vi "_TangoAttributeConfigEventGroupCreate.vi"(0 "error in":errorcluster) -> (1 "attribute config event ref":T1, 2 "error out":errorcluster)   [LabVIEW 2014, in "tango.lvlib"]
uses:
  tango.lvlib
  Common VIs/Typedefs/_AttributeConfigEventRef.ctl
  Common VIs/Typedefs/_AttributeInfo_t.ctl
  Common VIs/Typedefs/_AttributeAccess_t.ctl
  Common VIs/Typedefs/_AttributeFormat_t.ctl
  Common VIs/Typedefs/_TangoDataType_t.ctl
  Common VIs/Typedefs/_AttributeLevel_t.ctl
  tango_binding.so
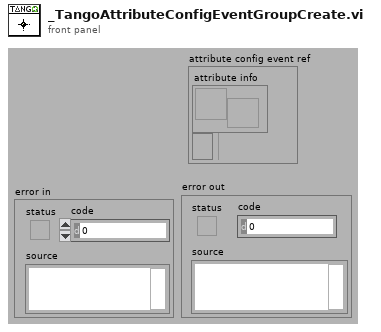
[diagram p1: front panel]
types:
  T1 = typedef "tango.lvlib/_AttributeConfigEventRef.ctl" = cluster{"attribute info":refnum<user-event>, "Event Registration Refnum":refnum<event-registration>}
  T2 = typedef "tango.lvlib/_AttributeInfo_t.ctl" = cluster{"device name":string, "attribute name":string, "r/w access":T3, "format":T4, "data type":T5, "level":T6, "label":string, "unit":string, "display format":string, "min value":string, "max value":string, "min alarm":string, "max alarm":string}
  T3 = typedef "tango.lvlib/_AttributeAccess_t.ctl" = enum16{"READ", "READ_WITH_WRITE", "WRITE", "READ_WRITE", "UNKNOWN_ACCESS_TYPE"}
  T4 = typedef "tango.lvlib/_AttributeFormat_t.ctl" = enum16{"SCALAR", "SPECTRUM", "IMAGE", "UNKNOWN_FORMAT"}
  T5 = typedef "tango.lvlib/_TangoDataType_t.ctl" = enum16{"VOID", "BOOLEAN", "SHORT", "LONG", "FLOAT", "DOUBLE", "USHORT", "ULONG", "STRING", "CHAR_ARRAY", "SHORT_ARRAY", "LONG_ARRAY", "FLOAT_ARRAY", "DOUBLE_ARRAY", "USHORT_ARRAY", "ULONG_ARRAY", "STRING_ARRAY", "LONG_STRING_ARRAY", "DOUBLE_STRING_ARRAY", "STATE", "CONST_STRING", "BOOLEAN_ARRAY", "UCHAR", "LONG64", "ULONG64", "LONG64_ARRAY", "ULONG64_ARRAY", "INT (not supported)", "ENCODED (not supported)", "ENUM", "PIPE_BLOB (not supported)", "STATE_ARRAY", "UNKNOW_DATA_TYPE"}
  T6 = typedef "tango.lvlib/_AttributeLevel_t.ctl" = enum16{"OPERATOR", "EXPERT", "UNKNOWN_LEVEL"}
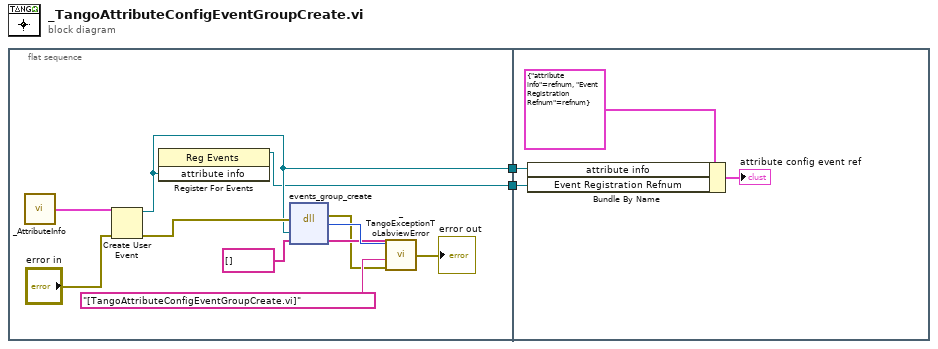
[diagram p0: block diagram]
diagram:
  n1 = flat-sequence {
    tunnel: [w5] -> w2
    tunnel: [w4] -> w1
    tunnel: w2 -> [w17]
    tunnel: w1 -> [w16]
    frame #0 {
      n2 = call "_AttributeInfo.vi"() -> ("attribute info"=w3:T2)  [unwired: 15 in]
      n3 = Create User Event(user event datatype=w3, error in="error in") -> (user event=w5:refnum<user-event>, error out=w12:errorcluster)
      n4 = register-events(w5) -> (reference out=w4:refnum<event-registration>)  [unwired: 2 in, 1 out]
      n5 = dll-call lib="tango_binding.*" fn="events_group_create"(error in=w12, "event refnum"=w5, "error_stack"=string[] []) -> (error out=w6:errorcluster, "return type"=w10:i32, "error_stack"=w9:string[])  [unwired: 3 in, 1 out]
      n6 = call "_TangoExceptionToLabviewError.vi"("error in"=w6, "location"="[TangoAttributeConfigEventGroupCreate.vi]", "error stack"=w9, "error code"=w10) -> ("error out"=→"error out":errorcluster)
    }
    frame #1 {
      n7 = Bundle By Name(cluster=T1 {"attribute info"=refnum, "Event Registration Refnum"=refnum} ("attribute config event ref"), "attribute info"=w17, "Event Registration Refnum"=w16) -> (→"attribute config event ref":T1)
    }
  }
